vi "Config Arc tolerance.vi"(0 "Arc tolerance (mm)":u32, 11 "error in (no error)":errorcluster) -> (15 "error out":errorcluster)   [LabVIEW 2024, in "GRBL 1.1.lvlib"]
doc: "Arc tolerance (mm): Sets the G2 and G3 arc tracing accuracy based on radial error. Beware: A very small value may effect performance."
uses:
  GRBL 1.1.lvlib
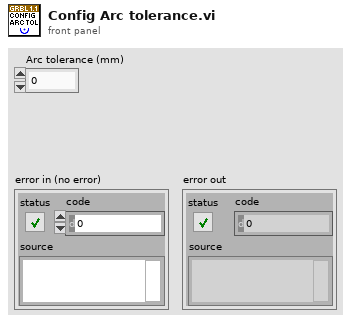
[diagram p1: front panel]
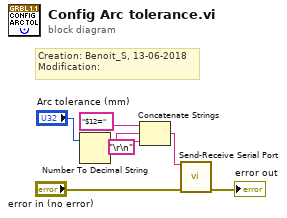
[diagram p0: block diagram]
diagram:
  # "Creation: Benoit_S, 13-06-2018\nModification:"
  n1 = Number To Decimal String(number="Arc tolerance (mm)") -> (decimal integer string=w5:string)  [unwired: 1 in]
  n2 = Concatenate Strings("$12=", w5, "\r\n") -> (w2:string)
  n3 = call "Send-Receive Serial Port.vi"("Data to write"=w2, "error in (no error)"="error in (no error)") -> ("error out"=→"error out":errorcluster)  [unwired: 12 in, 1 out]
